vi "DefineSingle.vi"(6 "Label":string="Custom" caption="Label (\"Custom\")", 9 "Error in":errorcluster caption="Error in (no error)", 10 "Custom description":string, 11 "Custom code":i32) -> ()   [LabVIEW 2017, in "GPError.lvlib"]
doc: "Dynamically defines a <B>Custom description</B> for <B>Custom code</B> effective in this entire LabVIEW session. This custom code can later be set on the error wire as either an error or a warning from anywhere in the LabVIEW session by using the SetError or SetWarning functions.\n\nThe optional <B>Label</B> (default \"Custom\") will be prepended the <B>Custom description</B> like this: \"<Label>:\\s\\s<Description>\" to conform to the format of the built-in descriptions. Wire an empty string to <B>Label</B> to omit the label entirely from the <B>Custom description</B> string.\n\nIf you define a <B>Custom code</B> that has already been defined once, <B>Custom description</B> will be appended to the existing array of descriptions for that <B>Custom code</B>. Any number of descriptions is supported for each code.\n\nIf you define a description for a <B>Custom code</B> that is a built-in error/warning code, then for the duration of this LabVIEW session this <B>Custom description</B> for that code will be appended to the built-in description(s).\n\nAll defined descriptions for a <B>Custom code</B> can be deleted again dynamically with the UndefineCustomCode function.\n\nThis VI runs only if there is no error on <B>Error in</B>.\n\nThis VI is polymorphic, accepting either a single description or an array of descriptions to define.\n\nSteen Schmidt\nGPower\n17/7 2013"
uses:
  GPError.lvlib
  FG/CustomErrorFGFunction.ctl
panel:
  # "Copyright © 2013\nSteen Schmidt, GPower\nSee enclosed license file for terms and conditions"
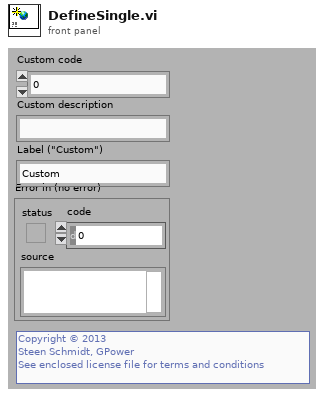
[diagram p1: front panel]
types:
  T1 = typedef "GPError.lvlib/CustomErrorFGFunction.ctl" = enum16{"Get custom descriptions", "Set custom code", "Unset custom code"}
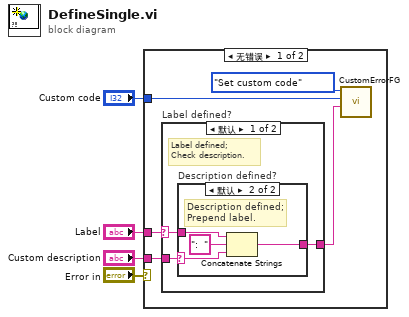
[diagram p0: block diagram]
diagram:
  n1 = case shown="无错误" "Error in" {
    tunnel: "Custom code" -> [w8 _]
    tunnel: "Custom description" -> [w6 _]
    tunnel: "Label" -> [w7 _]
    frame No Error {
      n2 = case "Label defined?" shown="默认" w7 {
        selector: w7 -> [w12 _]
        tunnel: w6 -> [w10 w17]
        tunnel: [w11 w17] -> w5
        frame Default {
          # "Label defined;\nCheck description."
          n3 = case "Description defined?" shown="默认" w10 {
            selector: w10 -> [_ w13]
            tunnel: w12 -> [_ w16]
            tunnel: [_ w14] -> w11
            frame "" {
              # "No description defined;\nOmit label as well."
            }
            frame Default {
              # "Description defined;\nPrepend label."
              n4 = Concatenate Strings(w16, ":  ", w13) -> (w14:string)
            }
          }
        }
        frame "" {
          # "No label defined;\nJust use description."
        }
      }
      n5 = call "CustomErrorFG.vi"("Custom description in"=w5, "Custom code"=w8, "Function"=CustomErrorFGFunction."Set custom code") -> ()  [unwired: 7 in, 2 out]
    }
    frame Error {
    }
  }
